vi "Control - PFI - Load Command.vi"(11 "Control Inputs":T1={"Engine Speed [RPM]"=0.0, "Engine Status"=enum."STALLED", "Load Control \nMode"=enum."No Governor", "dt(s)"=0.0, "Number of Cylinders"=0, "Engine Displacement [cc]"=0.0, "StoichAFR"=0.0, "Q.LHV Fuel [kJ/kg]"=0.0, "BattV PSU [V]"=0.0, "12V PSU [V]"=0.0, "5V PSU [V]"=0.0, "Pedal Position [%]"=0.0, "Oil Pressure [kPa]"=0.0, "Oil Temp [C]"=0.0, "Oil Level [%]"=0.0, "Engine Coolant Temp (ECT) [C]"=0.0, "Engine Coolant Pressure [kPa]"=0.0, "Rail Pressure [bar]"=0.0, "Fuel Pressure [kPa]"=0.0, "Fuel Temp [C]"=0.0, "Vacuum Pressure [kPa]"=0.0, "Throttle Position [%]"=0.0, "Cam1 Advance [CAD]"=0.0, "Cam2 Advance [CAD]"=0.0, "Cam3 Advance [CAD]"=0.0, "Cam4 Advance [CAD]"=0.0, "CA50 Control Output [CAD]"=[], "CA50 Control Output Valid"=[], "Intake Air Temp (IAT) [C]"=0.0, "Barometric Air Pressure [kPa]"=0.0, "Intake Air Rel. Humidity [%]"=0.0, "Mass Air Flow (MAF) [kg/hr]"=0.0, "Turbo Inlet Air Pressure [kPa]"=0.0, "Turbo Inlet Air Temp [C]"=0.0, "Turbo Outlet Air Pressure [kPa]"=0.0, "Turbo Outlet Air Temp [C]"=0.0, "CAC Outlet Pressure [kPa]"=0.0, "CAC Outlet Temp [C]"=0.0, "Intake Manifold Pressure (MAP) [kPa]"=0.0, "Intake Manifold Temp (MAT) [C]"=0.0, "Exhaust Manifold Pressure [kPa]"=0.0, "Exhaust Manifold Temp [C]"=0.0, "HighP EGR Cooler Outlet Pressure [kPa]"=0.0, "HighP EGR Cooler Outlet Temp [C]"=0.0, "HighP EGR Differential Pressure [kPa]"=0.0, "HighP EGR Valve Position [%]"=0.0, "Turbo Outlet Exhaust Pressure [kPa]"=0.0, "Turbo Outlet Exhaust Temp [C]"=0.0, "VGT Position 1 [%]"=0.0, "VGT Position 2 [%]"=0.0, "Turbo Speed 1 [RPM]"=0.0, "Turbo Speed 2 [RPM]"=0.0, "LowP EGR Differential Pressure [kPa]"=0.0, "LowP EGR Valve Position [%]"=0.0, "UEGO1Lambda"=0.0, "UEGO1_Hot"=FALSE, "UEGO2Lambda"=0.0, "UEGO2_Hot"=FALSE, "Knock Intensity"=[], "Knock"=[]} {"Knock Intensity" format="%.2f"; "CA50 Control Output [CAD]" format="%.2f"; "Exhaust Manifold Temp [C]" format="%#_6f"; "UEGO2Lambda" format="%.2f"; "Intake Manifold Temp (MAT) [C]" format="%#_6f"; "UEGO1Lambda" format="%.2f"}) -> (1 "Integral Governor Control [%]":sgl, 2 "Rapid (P+D) Governor Control [%]":sgl, 3 "IMEP Desired [bar]":sgl)   [LabVIEW 2015, in "ECS-RT.lvlib"]
uses:
  ECS-RT.lvlib
  Typedefs/Control Inputs/Control Inputs.ctl
  Typedefs/EPT/Engine Status.ctl
  Typedefs/MISC/Load Control Mode.ctl
  ECS-Shared.lvlib
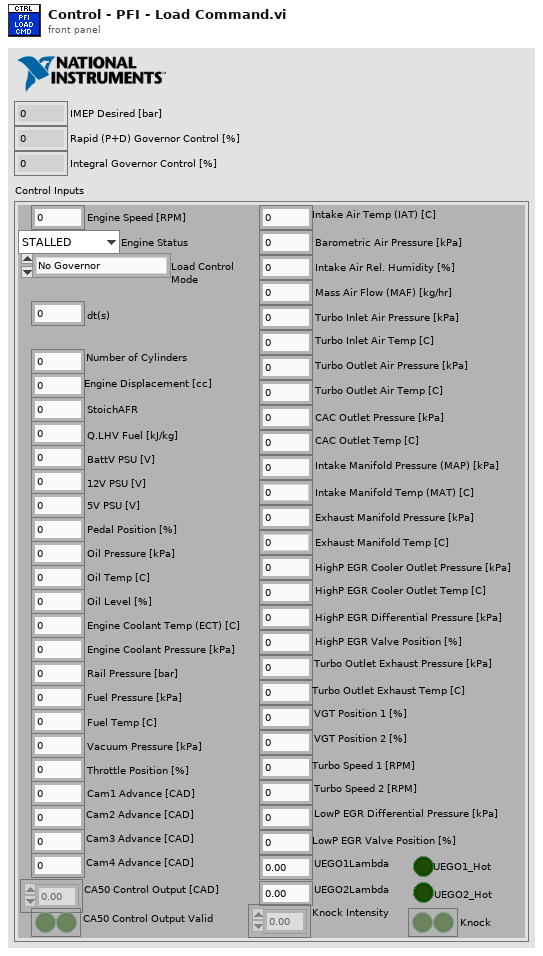
[diagram p1: front panel]
types:
  T1 = typedef "ECS-Shared.lvlib/Control Inputs.ctl" = cluster{"Engine Speed [RPM]":sgl, "Engine Status":T2, "Load Control \nMode":T3, "dt(s)":sgl, "Number of Cylinders":u8, "Engine Displacement [cc]":sgl, "StoichAFR":sgl, "Q.LHV Fuel [kJ/kg]":sgl, "BattV PSU [V]":sgl, "12V PSU [V]":sgl, "5V PSU [V]":sgl, "Pedal Position [%]":sgl, "Oil Pressure [kPa]":sgl, "Oil Temp [C]":sgl, "Oil Level [%]":sgl, "Engine Coolant Temp (ECT) [C]":sgl, "Engine Coolant Pressure [kPa]":sgl, "Rail Pressure [bar]":sgl, "Fuel Pressure [kPa]":sgl, "Fuel Temp [C]":sgl, "Vacuum Pressure [kPa]":sgl, "Throttle Position [%]":sgl, "Cam1 Advance [CAD]":sgl, "Cam2 Advance [CAD]":sgl, "Cam3 Advance [CAD]":sgl, "Cam4 Advance [CAD]":sgl, "CA50 Control Output [CAD]":sgl[], "CA50 Control Output Valid":bool[], "Intake Air Temp (IAT) [C]":sgl, "Barometric Air Pressure [kPa]":sgl, "Intake Air Rel. Humidity [%]":sgl, "Mass Air Flow (MAF) [kg/hr]":sgl, "Turbo Inlet Air Pressure [kPa]":sgl, "Turbo Inlet Air Temp [C]":sgl, "Turbo Outlet Air Pressure [kPa]":sgl, "Turbo Outlet Air Temp [C]":sgl, "CAC Outlet Pressure [kPa]":sgl, "CAC Outlet Temp [C]":sgl, "Intake Manifold Pressure (MAP) [kPa]":sgl, "Intake Manifold Temp (MAT) [C]":sgl, "Exhaust Manifold Pressure [kPa]":sgl, "Exhaust Manifold Temp [C]":sgl, "HighP EGR Cooler Outlet Pressure [kPa]":sgl, "HighP EGR Cooler Outlet Temp [C]":sgl, "HighP EGR Differential Pressure [kPa]":sgl, "HighP EGR Valve Position [%]":sgl, "Turbo Outlet Exhaust Pressure [kPa]":sgl, "Turbo Outlet Exhaust Temp [C]":sgl, "VGT Position 1 [%]":sgl, "VGT Position 2 [%]":sgl, "Turbo Speed 1 [RPM]":sgl, "Turbo Speed 2 [RPM]":sgl, "LowP EGR Differential Pressure [kPa]":sgl, "LowP EGR Valve Position [%]":sgl, "UEGO1Lambda":sgl, "UEGO1_Hot":bool, "UEGO2Lambda":sgl, "UEGO2_Hot":bool, "Knock Intensity":sgl[], "Knock":bool[]}
  T2 = typedef "ECS-Shared.lvlib/Engine Status.ctl" = enum16{"OFF", "STALLED", "CRANKING", "RUNNING", "ACCEL", "DECEL", "SAFE"}
  T3 = typedef "ECS-Shared.lvlib/Load Control Mode.ctl" = enum16{"No Governor", "Min Speed Governor", "Max Speed Governor"}
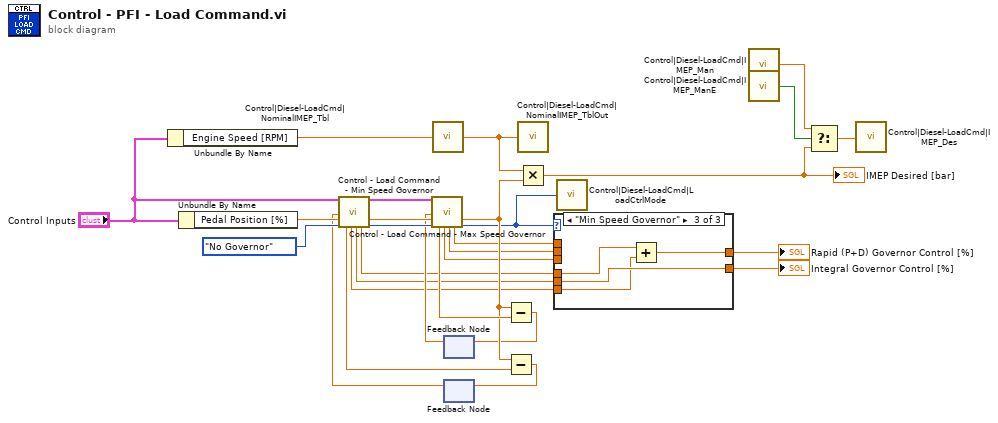
[diagram p0: block diagram]
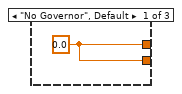
[diagram p2: hidden frame]
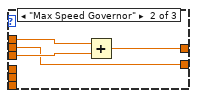
[diagram p3: hidden frame]
diagram:
  n1 = Unbundle By Name("Control Inputs") -> ("Engine Speed [RPM]"=w28:sgl)
  n2 = Unbundle By Name("Control Inputs") -> ("Pedal Position [%]"=w25:sgl)
  n3 = call "Control|Diesel-LoadCmd|NominalIMEP_Tbl"("X Index"=w28) -> ("Y"=w27:sgl)
  n4 = feedback #1() -> (w16:sgl)  [unwired: 1 in]
  n5 = feedback #2() -> (w14:sgl)  [unwired: 1 in]
  n6 = call "Control - Load Command - Min Speed Governor.vi"("Control Inputs"="Control Inputs", "BeatbackDiff"=w14, "Pedal In"=w25, "Load Control Mode In"=Load_Control_Mode."No Governor") -> ("Governor Output"=w18:sgl, "PEffort"=w8:sgl, "IEffort"=w9:sgl, "DEffort"=w10:sgl, "Control Inputs"=w21:T1, "Pedal Out"=w24:sgl, "Load Control Mode Out"=w23:T3)  [unwired: 9 in]
  n7 = call "Control - Load Command - Max Speed Governor.vi"("Control Inputs"=w21, "BeatbackDiff"=w16, "Pedal In"=w24, "Load Control Mode In"=w23) -> ("Governor Output"=w20:sgl, "PEffort"=w11:sgl, "IEffort"=w12:sgl, "DEffort"=w13:sgl, "Pedal Out"=w19:sgl, "Load Control Mode Out"=w1:T3)  [unwired: 9 in, 1 out]
  n8 = Subtract(x=w19, y=w20) -> (x-y=w17:sgl)
  n9 = feedback-in #1(w17) -> ()
  n10 = Subtract(x=w19, y=w18) -> (x-y=w15:sgl)
  n11 = feedback-in #2(w15) -> ()
  n12 = call "Control|Diesel-LoadCmd|NominalIMEP_TblOut"("Value"=w27) -> ()
  n13 = Multiply(x=w27, y=w19) -> (x*y=w3:sgl)
  "IMEP Desired [bar]" <- w3
  n14 = case shown="\"Min Speed Governor\"" w1 {
    tunnel: w13 -> [_ w33 _]
    tunnel: w12 -> [_ w30 _]
    tunnel: w11 -> [_ w32 _]
    tunnel: w10 -> [_ _ w34]
    tunnel: w9 -> [_ _ w36]
    tunnel: w8 -> [_ _ w35]
    tunnel: [w29 w31 w37] -> w7
    tunnel: [w29 w30 w36] -> w6
    frame "No Governor", Default {
      w29 = sgl 0.0 ("Rapid (P+D) Governor Control")
    }
    frame "Max Speed Governor" {
      n15 = Add(x=w33, y=w32) -> (x+y=w31:sgl)
    }
    frame "Min Speed Governor" {
      n16 = Add(x=w34, y=w35) -> (x+y=w37:sgl)
    }
  }
  "Rapid (P+D) Governor Control [%]" <- w7
  "Integral Governor Control [%]" <- w6
  n17 = call "Control|Diesel-LoadCmd|LoadCtrlMode"("Value"=w1) -> ()
  n18 = call "Control|Diesel-LoadCmd|IMEP_Man"() -> ("Value"=w5:sgl)
  n19 = call "Control|Diesel-LoadCmd|IMEP_ManE"() -> ("Value"=w4:bool)
  n20 = Select(t=w5, s=w4, f=w3) -> (s? t:f=w2:sgl)
  n21 = call "Control|Diesel-LoadCmd|IMEP_Des"("Value"=w2) -> ()
